vi "New.vi"(8 "error in (no error)":errorcluster, 10 "Private Data":T1, 11 "Skeleton in":refnum<class "Skeleton.lvclass">) -> (0 "error out":errorcluster, 3 "Skeleton out":refnum<class "Skeleton.lvclass">)   [LabVIEW 2016, in "Skeleton.lvlib" / "Skeleton.lvclass"]
uses:
  Skeleton.lvclass
  Private Data.ctl
  Skeleton.lvclass/Skeleton.ctl
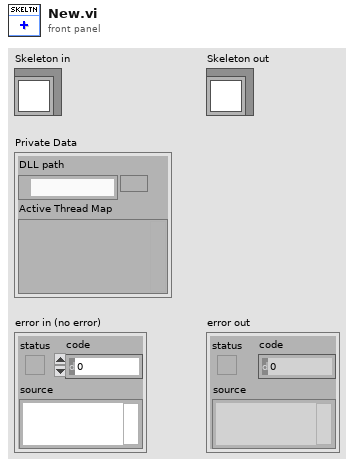
[diagram p1: front panel]
types:
  T1 = typedef "Skeleton.lvlib/Skeleton.lvclass/Private Data.ctl" = cluster{"DLL path":path, "Active Thread Map":variant}
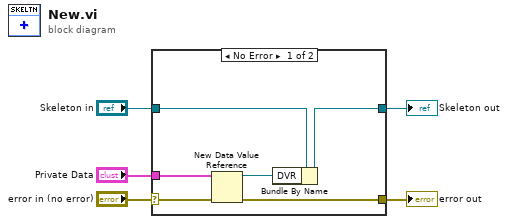
[diagram p0: block diagram]
diagram:
  n1 = case shown="No Error" "error in (no error)" {
    selector: "error in (no error)" -> [w11 w13]
    tunnel: [w10 w13] -> w4
    tunnel: [w6 w12] -> w2
    tunnel: "Skeleton in" -> [w7 w12]
    tunnel: "Private Data" -> [w9 _]
    frame No Error {
      n2 = New Data Value Reference(data value=w9, error in=w11) -> (data value reference=w8:refnum<data-value>, error out=w10:errorcluster)
      n3 = Bundle By Name(cluster=w7, "DVR"=w8) -> (w6:refnum<class "Skeleton.lvclass">)
    }
    frame Error {
    }
  }
  "error out" <- w4
  "Skeleton out" <- w2
